vi "Thermometers.vi"() -> ()   [LabVIEW 2014]
panel:
  in  "stop":bool
  out "Degree F":dbl
  out "Thermometer F":dbl(slide) caption="Celsius" scale=0.0..100.0
  out "Thermometer C":dbl(slide) caption="Fahrenheit" scale=0.0..100.0
  in  "Degree C":dbl
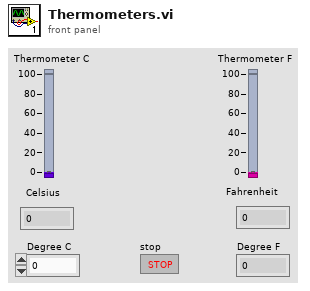
[diagram p1: front panel]
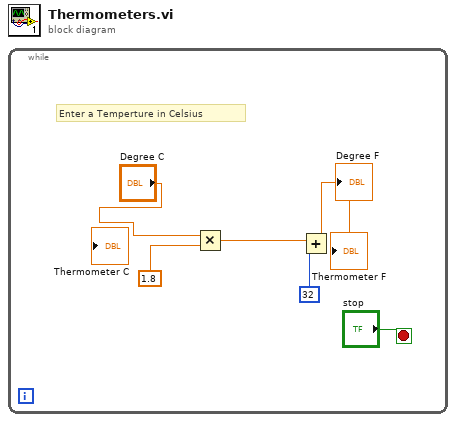
[diagram p0: block diagram]
diagram:
  n1 = while {
    stop <- "stop" stop-if-true
    # "Enter a Temperture in Celsius"
    n2 = Multiply(x="Degree C", y=1.8) -> (x*y=w5:dbl)
    n3 = Add(x=w5, y=32) -> (x+y=→"Degree F" →"Thermometer F":dbl)
  }
